vi "Table Load for 工單號碼.vi"(8 "error in (no error)":errorcluster, 11 "appended path":path) -> (3 "EnfMeasureTable":cluster{"Table Control":string[][]}[](array[cluster]))   [LabVIEW 2019]
uses:
  <vilib>/Utility/sysdir.llb/System Directory Type.ctl
  Ctrl/Table Save.ctl
  <vilib>/Utility/xml.llb/Read From XML File(string).vi
  f3f038a6-a736-4945-a354-3d30d0424a0a.vi
  a2377119-9521-4aef-8846-be355f26f971.vi
  <vilib>/Utility/xml.llb/Write to XML File(string).vi
panel:
  in  "EnfMeasureTable 5":cluster{"Table Control":string[][]}[](array[cluster])
  out "EnfMeasureTable 3":cluster{"Table Control":string[][]}[](array[cluster])
  out "value":cluster{"Table Control":string[][]}[](array[cluster])
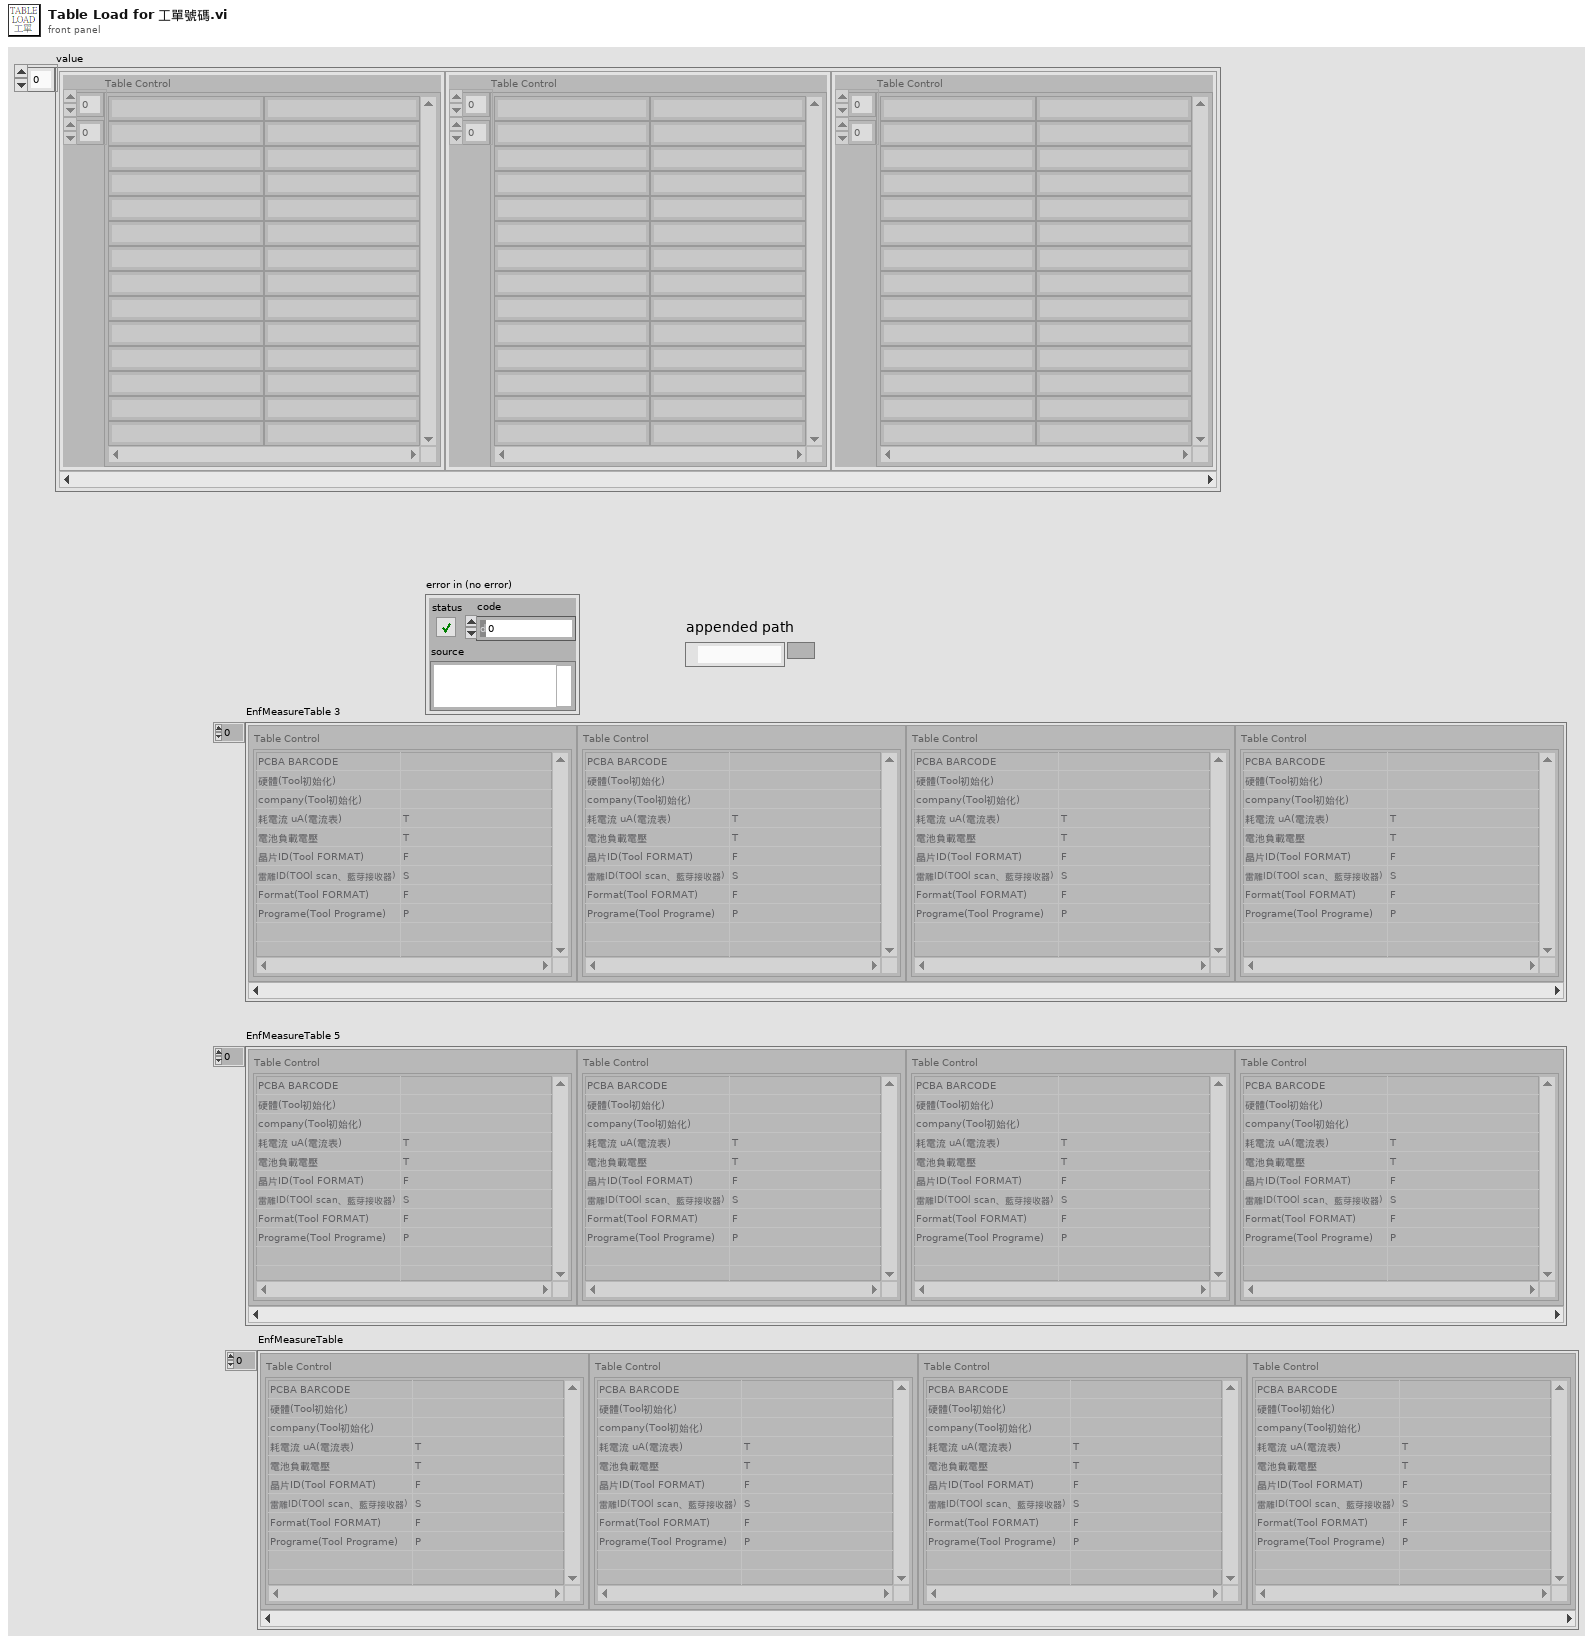
[diagram p1: front panel]
types:
  T1 = typedef "Table Save.ctl" = enum16{"initial", "Add", "Write", "Replace", "Delete", "REad", "RedTable", "Load"}
  T2 = typedef "System Directory Type.ctl" = i32
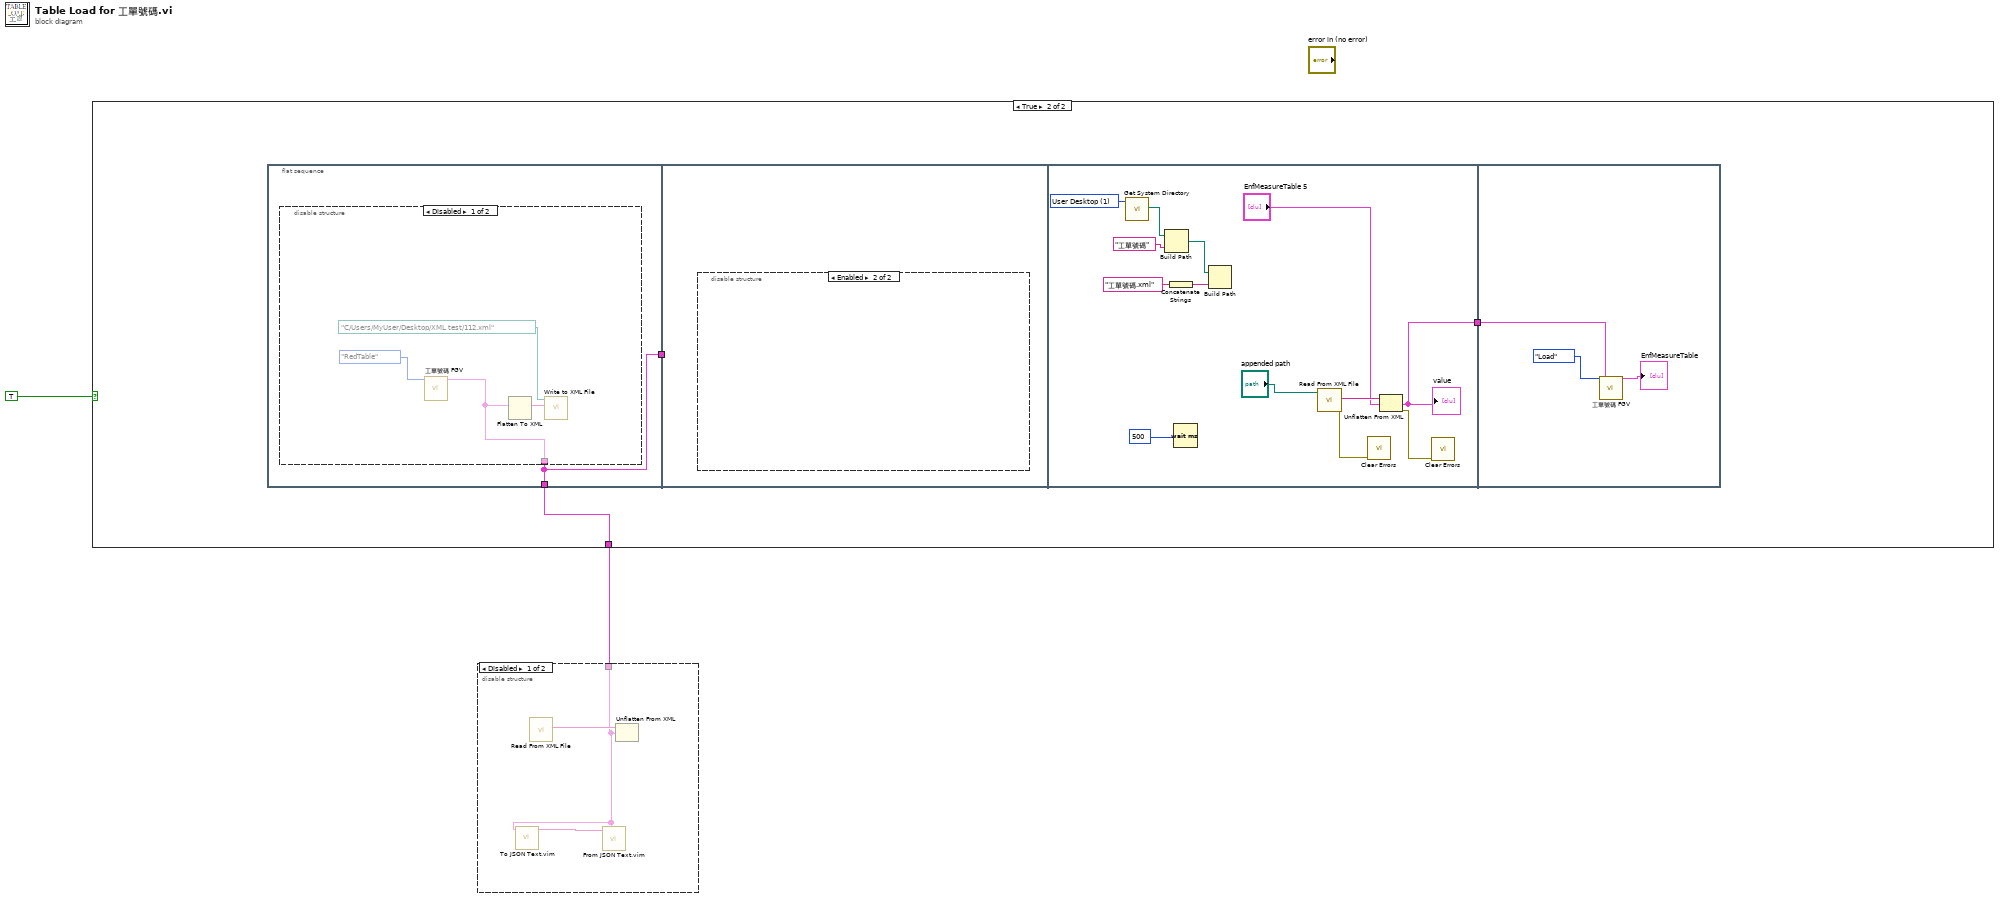
[diagram p0: block diagram]
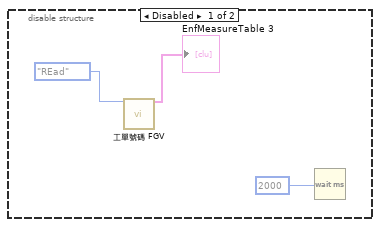
[diagram p4: hidden frame]
diagram:
  n1 = case shown="True" TRUE {
    tunnel: [_ w4] -> w2
    frame False {
    }
    frame True {
      n2 = flat-sequence {
        tunnel: [w6] -> w4
        tunnel: [w6] -> w5
        tunnel: w5 -> [_]
        tunnel: [w23] -> w3
        tunnel: w3 -> [w27]
        frame #0 {
          n3 = disable-structure shown="Disabled" {
            disable-tunnel: [w7 _] -> w6
            frame Disabled {
              n4 = call "工單號碼 FGV.vi"("Action"=Table_Save."RedTable") -> ("Total Table"=w7:cluster{"Table Control":string[][]}[])  [unwired: 11 in, 7 out]
              n5 = Flatten To XML(anything=w7) -> (xml string=w10:string)
              n6 = call-poly <vilib>:"Write to XML File.vi"("XML Input"=w10, "XML File Path"=path "C:/Users/MyUser/Desktop/XML test/112.xml") -> ()  [unwired: 7 in, 3 out]
            }
            frame Enabled {
            }
          }
        }
        frame #1 {
          n7 = disable-structure shown="Enabled" {
            frame Disabled {
              n8 = call "工單號碼 FGV.vi"("Action"=Table_Save."REad") -> ("Total Table"=→"EnfMeasureTable 3":cluster{"Table Control":string[][]}[])  [unwired: 11 in, 7 out]
              n9 = Wait (ms)(milliseconds to wait=2000) -> ()  [unwired: 1 out]
            }
            frame Enabled {
            }
          }
        }
        frame #2 {
          w20 = T2 1 items=["User Home"=0, "User Desktop"=1, "User Documents"=2, "User Application Data"=3, "User Preferences"=4, "User Temporary"=5, "Public Documents"=6, "Public Application Data"=7, "Public Preferences"=8, "Public Cache"=13, "System Core Libraries"=9, "System Installed Libraries"=10, "Application Files"=11, "Boot Volume Root"=12] ("system directory type")
          n10 = call <vilib>:"Get System Directory.vi"("system directory type"=w20) -> ("system directory"=w18:path)  [unwired: 10 in]
          n11 = Build Path(base path=w18, name or relative path="工單號碼") -> (appended path=w16:path)
          n12 = Concatenate Strings("工單號碼.xml" ("string")) -> (w17:string)
          n13 = Wait (ms)(milliseconds to wait=500) -> ()  [unwired: 1 out]
          n14 = Build Path(base path=w16, name or relative path=w17) -> ()  [unwired: 1 out]
          n15 = call-poly <vilib>:"Read From XML File.vi"("XML File Path"="appended path") -> ("error out"=w21:errorcluster, "XML Elements"=w26:string)  [unwired: 8 in, 1 out]
          n16 = call <vilib>:"Clear Errors.vi"("error in (no error)"=w21) -> ()  [unwired: 5 in, 2 out]
          n17 = Unflatten From XML(xml string=w26, type="EnfMeasureTable 5") -> (value=w23:cluster{"Table Control":string[][]}[], error out=w22:errorcluster)  [unwired: 1 in]
          "value" <- w23
          n18 = call <vilib>:"Clear Errors.vi"("error in (no error)"=w22) -> ()  [unwired: 5 in, 2 out]
        }
        frame #3 {
          n19 = call "工單號碼 FGV.vi"("Action"=Table_Save."Load", "Table Load"=w27) -> ("Total Table"=→"EnfMeasureTable":cluster{"Table Control":string[][]}[])  [unwired: 10 in, 7 out]
        }
      }
    }
  }
  n20 = disable-structure shown="Disabled" {
    disable-tunnel: w2 -> [w30 _]
    frame Disabled {
      n21 = call "To JSON Text.vim"("Anything"=w30) -> ("<JSON>"=w32:string)  [unwired: 9 in, 1 out]
      n22 = call-poly <vilib>:"Read From XML File.vi"() -> ("XML Elements"=w31:string)  [unwired: 9 in, 2 out]
      n23 = call "From JSON Text.vim"("Data Type and Default Value"=w30, "JSON"=w32) -> ()  [unwired: 8 in, 2 out]
      n24 = Unflatten From XML(xml string=w31, type=w30) -> ()  [unwired: 1 in, 2 out]
    }
    frame Enabled {
    }
  }
